vi "Dynamic.vi"() -> ()   [LabVIEW 2018]
panel:
  in  "Enum":enum16{"Sine", "Square", "Triangle"}(ring)
  in  "stop":bool
  out "Waveform Graph":dynamicdata(graph)
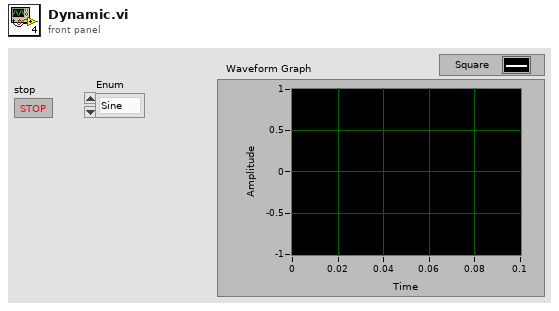
[diagram p1: front panel]
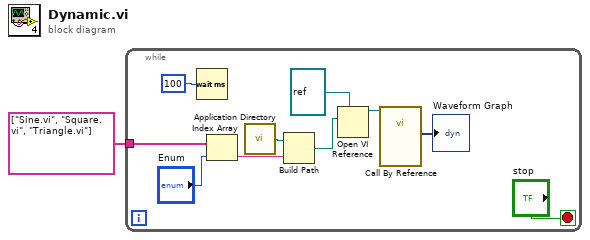
[diagram p0: block diagram]
diagram:
  n1 = while {
    tunnel: string[] ["Sine.vi", "Square.vi", "Triangle.vi"] -> [w8]
    stop <- "stop" stop-if-true
    n2 = Wait (ms)(milliseconds to wait=u32 100) -> ()  [unwired: 1 out]
    n3 = Index Array(array=w8, index="Enum") -> (element=w6:string)
    n4 = call <vilib>:"Application Directory.vi"() -> ("Application Directory"=w9:path)
    n5 = Build Path(base path=w9, name or relative path=w6) -> (appended path=w5:path)
    n6 = Open VI Reference(type specifier VI Refnum (for type only)=refnum<vi> refnum, vi path=w5) -> (vi reference=w4:refnum<vi>)  [unwired: 4 in, 1 out]
    n7 = call-by-ref "?"(reference=w4) -> ("Sine"=→"Waveform Graph":dynamicdata)  [unwired: 12 in, 2 out]
  }
